vi "ModelShiftingLatency.vi"(1 "Swerve_Solenoid_Output":T1) -> (0 "Actual State":bool)   [LabVIEW 2019]
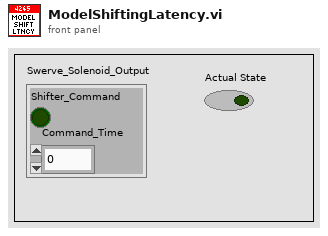
[diagram p1: front panel]
types:
  T1 = cluster{"Shifter_Command":bool, "Command_Time":u32}
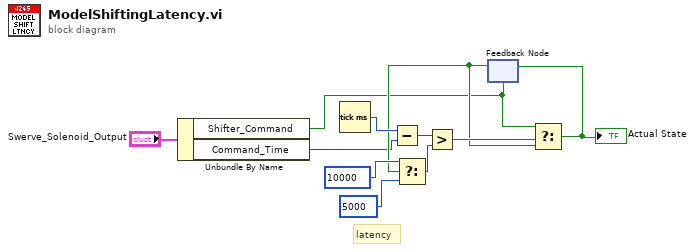
[diagram p0: block diagram]
diagram:
  # "latency"
  n1 = Unbundle By Name("Swerve_Solenoid_Output") -> ("Shifter_Command"=w2:bool, "Command_Time"=w3:u32)
  n2 = Tick Count (ms)() -> (millisecond timer value=w10:u32)
  n3 = Subtract(x=w10, y=w3) -> (x-y=w9:u32)
  n4 = feedback #1(w2) -> (w4:bool)
  n5 = Select(t=u32 10000 ("x"), s=w4, f=u32 5000) -> (s? t:f=w8:u32)
  n6 = Greater?(x=w9, y=w8) -> (0:w5:bool)
  n7 = Select(t=w2, s=w5, f=w4) -> (s? t:f=w11:bool)
  "Actual State" <- w11
  n8 = feedback-in #1(w11) -> ()
